vi "SubVI RX IQ Waveform.vi"(8 "错误输入":errorcluster, 11 "接收IQ波形":cluster{"t0":dbl, "dt":dbl, "Y":cdb[]}) -> (0 "错误输出":errorcluster, 4 "I":waveform(dbl), 6 "Q":waveform(dbl))   [LabVIEW 2015]
uses:
  <vilib>/addons/Modulation/niAMT.lvlib
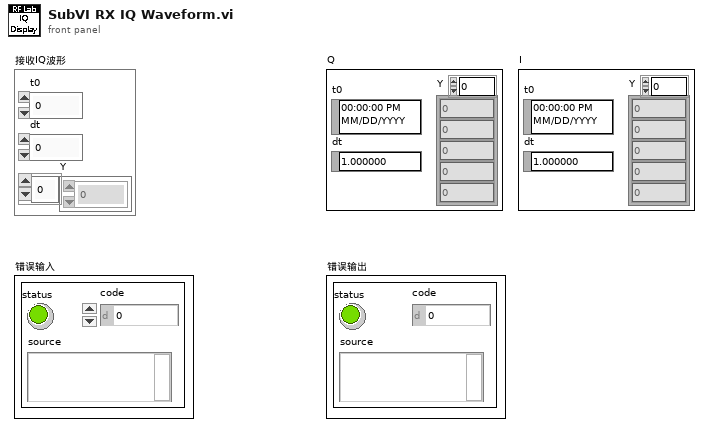
[diagram p1: front panel]
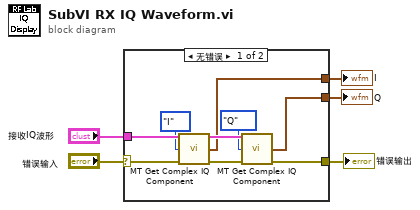
[diagram p0: block diagram]
diagram:
  n1 = case shown="无错误" "错误输入" {
    selector: "错误输入" -> [w6 w15]
    tunnel: "接收IQ波形" -> [w14 _]
    tunnel: [w12 w15] -> w4
    tunnel: [w8 _] -> w3
    tunnel: [w7 _] -> w2
    frame No Error {
      n2 = call <vilib>:"MT Get Complex IQ Component.vi"("IQ data (complex) in"=w14, "component choice"=enum16{"I", "Q", "Magnitude", "Phase"}."I", "error in (no error)"=w6) -> ("IQ data (complex) out"=w13:cluster{"t0":dbl, "dt":dbl, "Y":cdb[]}, "CE component"=w8:waveform(dbl), "error out"=w9:errorcluster)  [unwired: 10 in]
      n3 = call <vilib>:"MT Get Complex IQ Component.vi"("IQ data (complex) in"=w13, "component choice"=enum16{"I", "Q", "Magnitude", "Phase"}."Q", "error in (no error)"=w9) -> ("CE component"=w7:waveform(dbl), "error out"=w12:errorcluster)  [unwired: 10 in, 1 out]
    }
    frame Error {
    }
  }
  "错误输出" <- w4
  "I" <- w3
  "Q" <- w2
